vi "prelookup_cmd.vi"(11 "Command":string) -> (1 "refnum name out":string, 2 "index":u8, 3 "arguments":string[](array[string]))   [LabVIEW 2014]
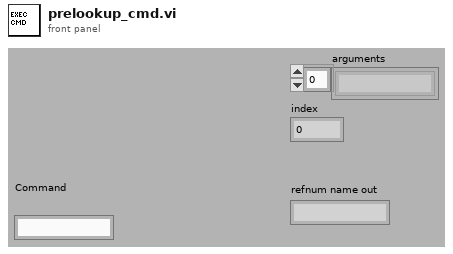
[diagram p1: front panel]
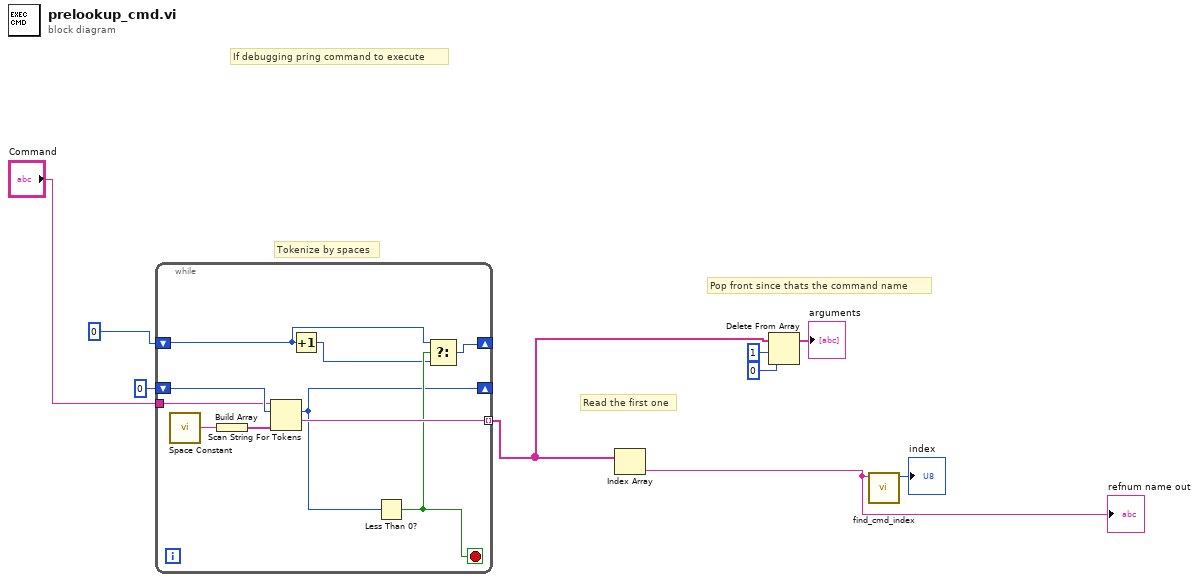
[diagram p0: block diagram]
diagram:
  # "If debugging pring command to execute"
  # "Pop front since thats the command name"
  # "Read the first one"
  # "Tokenize by spaces"
  n1 = while {
    shift-right: [w10] -> _
    shift-left: 0 ("offset past token") -> [w19]
    tunnel: "Command" -> [w18]
    tunnel: [w17] -> w6 mode=indexing
    shift-right: [w13] -> _
    shift-left: u8 0 -> [w15]
    stop <- w16 stop-if-true
    n2 = call <vilib>:"Space Constant.vi"() -> ("String"=w12:string)
    n3 = Build Array(w12) -> (w11:string[])
    n4 = Scan String For Tokens(6:w11, 8:w19, 9:w18) -> (1:w17:string, 2:w10:i32)  [unwired: 5 out]
    n5 = Increment(x=w15) -> (x+1=w14:u8)
    n6 = Less Than 0?(x=w10) -> (x < 0?=w16:bool)
    n7 = Select(t=w15, s=w16, f=w14) -> (s? t:f=w13:u8)
  }
  n8 = Index Array(array=w6) -> (element=w1:string)  [unwired: 1 in]
  "refnum name out" <- w1
  n9 = Delete From Array(array=w6, length=1, index=0) -> (array with subset deleted=→"arguments":string[])  [unwired: 1 out]
  n10 = call "find_cmd_index.vi"("cmd_name"=w1) -> ("index"=→"index":u8)  [unwired: 10 in]
